vi "setnag_o2_gauge_subVI.vi"(10 "setnag info in":T1) -> (1 "Cluster":cluster{"Numeric Control":dbl}, 2 "Numeric Control out":dbl, 3 "Array":dbl[](array[numeric]), 5 "String":string)   [LabVIEW 2014]
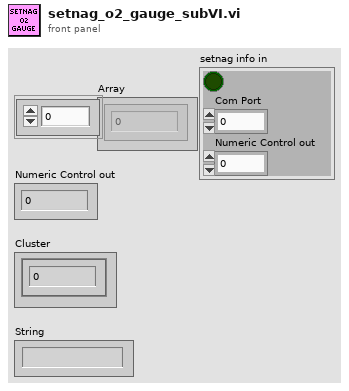
[diagram p1: front panel]
types:
  T1 = cluster{bool, "Com Port":i32, "Numeric Control out":dbl}
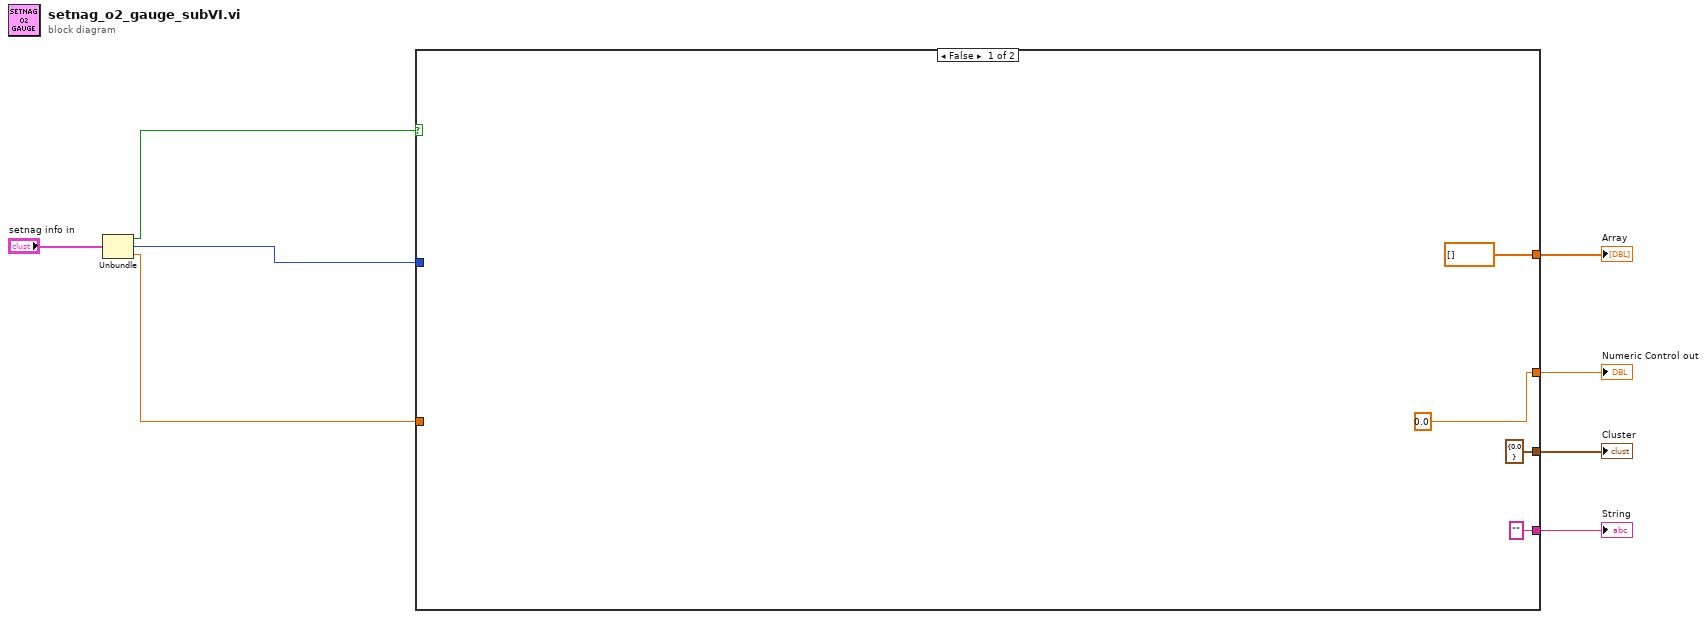
[diagram p0: block diagram]
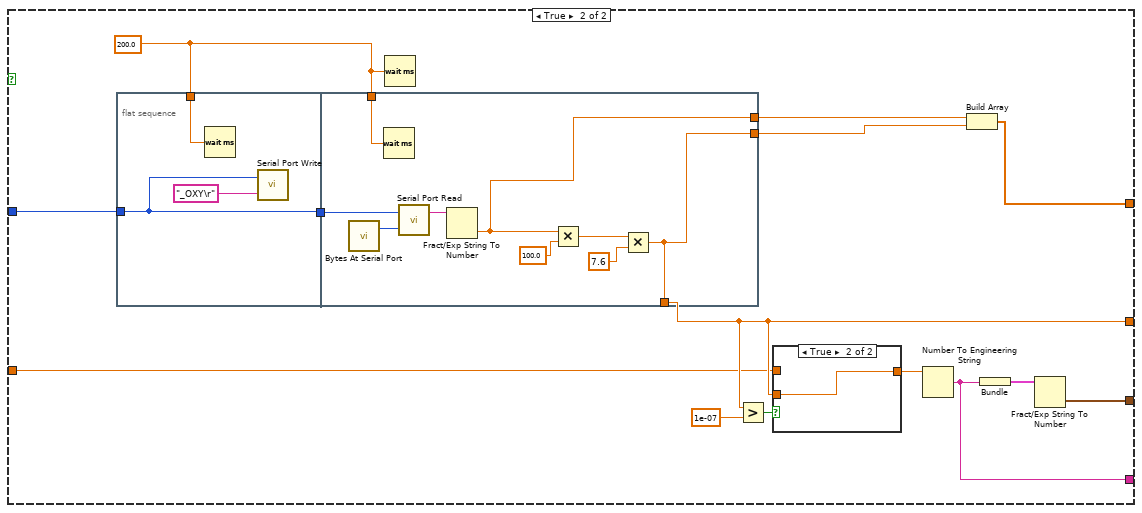
[diagram p2: hidden frame]
diagram:
  n1 = Unbundle("setnag info in") -> (w3:bool, "Com Port"=w2:i32, "Numeric Control out"=w1:dbl)
  n2 = case shown="False" w3 {
    tunnel: [cluster{dbl} {0.0} w25] -> w8
    tunnel: [dbl[] [] w24] -> w7
    tunnel: ["" w20] -> w6
    tunnel: w2 -> [_ w19]
    tunnel: [0.0 w18] -> w5
    tunnel: w1 -> [_ w17]
    frame False {
    }
    frame True {
      w21 = 200.0 ("Numeric Control in")
      n3 = flat-sequence {
        tunnel: [w29] -> w26
        tunnel: w21 -> [w31]
        tunnel: w19 -> [w29]
        tunnel: w26 -> [w35]
        tunnel: w21 -> [w39]
        tunnel: [w32] -> w18
        tunnel: [w34] -> w22
        tunnel: [w32] -> w23
        frame #0 {
          n4 = Wait (ms)(milliseconds to wait=w31) -> ()  [unwired: 1 out]
          n5 = call <vilib>:"Serial Port Write.vi"("string to write"="_OXY\r" ("O2 partial press"), "port number"=w29) -> ()  [unwired: 1 out]
        }
        frame #1 {
          n6 = call <vilib>:"Bytes At Serial Port.vi"() -> ("byte count"=w40:u32)  [unwired: 1 in, 1 out]
          n7 = Wait (ms)(milliseconds to wait=w39) -> ()  [unwired: 1 out]
          n8 = call <vilib>:"Serial Port Read.vi"("requested byte count"=w40, "port number"=w35) -> ("string read"=w38:string)  [unwired: 1 out]
          n9 = Fract/Exp String To Number(string=w38) -> (number=w34:dbl)  [unwired: 3 in, 1 out]
          n10 = Multiply(x=w34, y=100.0) -> (x*y=w33:dbl)
          n11 = Multiply(x=w33, y=7.6) -> (x*y=w32:dbl)
        }
      }
      n12 = Wait (ms)(milliseconds to wait=w21) -> ()  [unwired: 1 out]
      n13 = Greater?(x=w18, y=1e-07) -> (0:w15:bool)
      n14 = case shown="True" w15 {
        tunnel: [w27 w28] -> w16
        tunnel: w18 -> [_ w28]
        tunnel: w17 -> [w27 _]
        frame False {
        }
        frame True {
        }
      }
      n15 = Number To Engineering String(4:w16) -> (0:w20:string)  [unwired: 3 in]
      n16 = Build Array(w22, w23) -> (w24:dbl[])
      n17 = Bundle(w20) -> (w13:cluster{string})  [unwired: 1 in]
      n18 = Fract/Exp String To Number(string=w13) -> (number=w25:cluster{dbl})  [unwired: 3 in, 1 out]
    }
  }
  "Cluster" <- w8
  "Array" <- w7
  "String" <- w6
  "Numeric Control out" <- w5
